vi "analyzepreLabel.vi"(0 "input_str_preLabel":string="L7KQF003-SD-R1510100004", 1 "input_int_SNNum":i32) -> (2 "show_bool_legal":bool, 3 "show_time_date":timestamp, 4 "show_str_message":string)   [LabVIEW 2011]
panel:
  out "midVar_str_yymmdd":string
  # "L7KQF003-SD-R1510100004\n    151010\nLR151010000001\n    101000\nLR15"
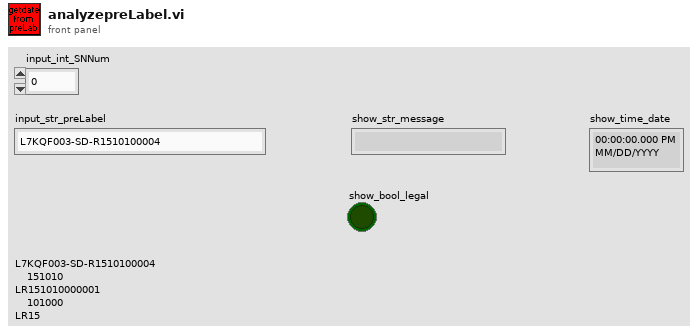
[diagram p1: front panel]
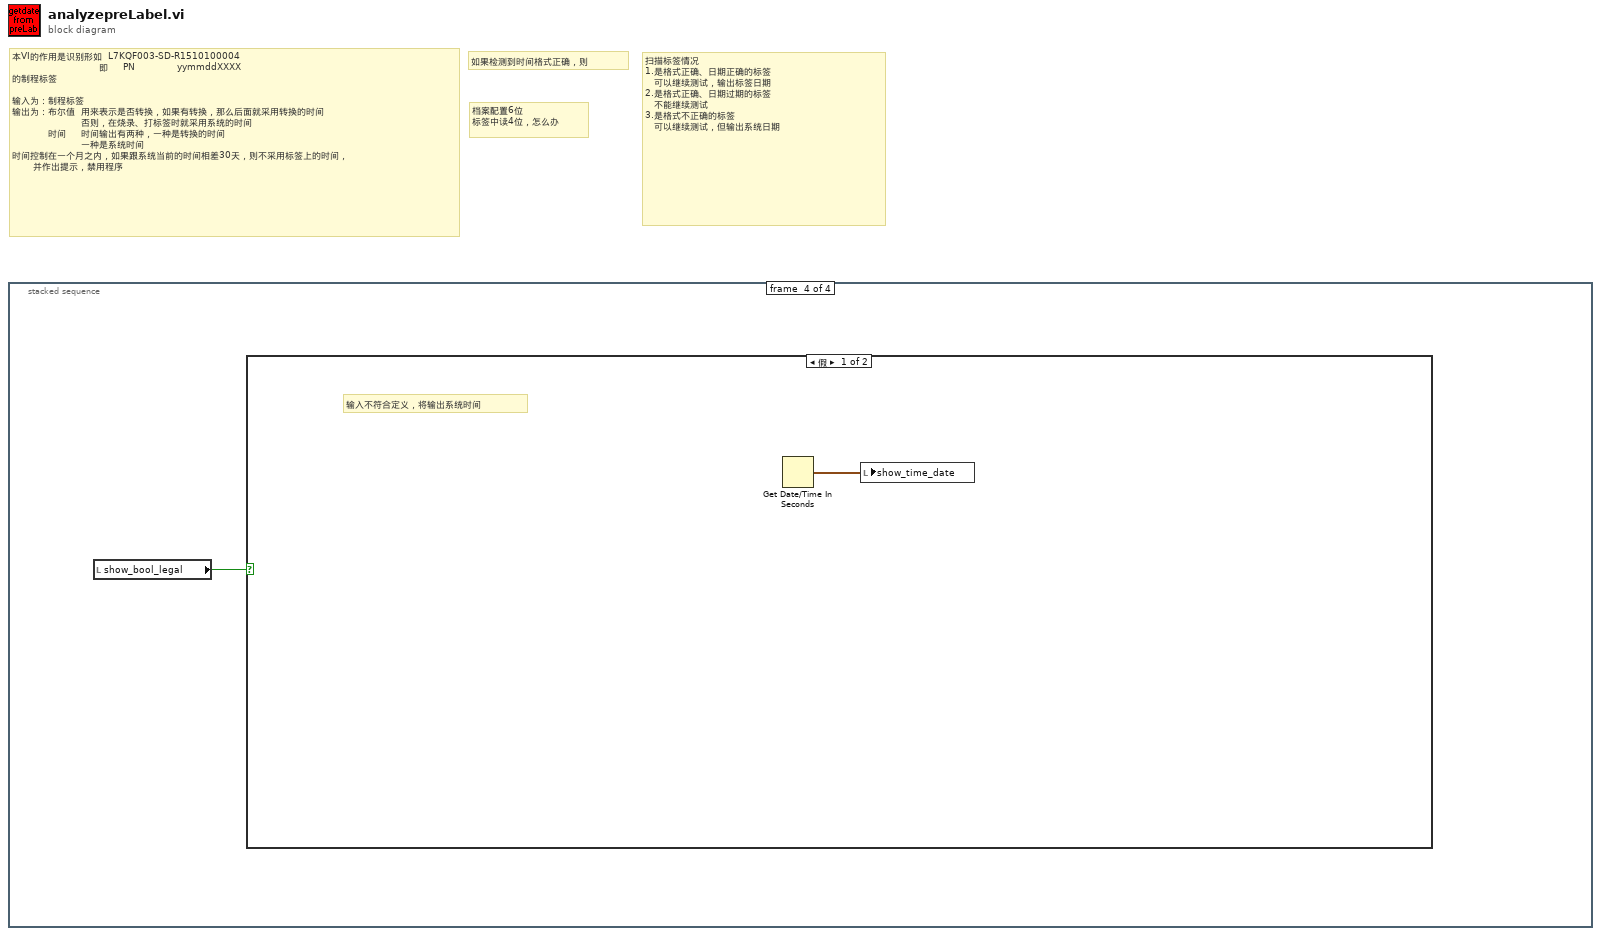
[diagram p0: block diagram]
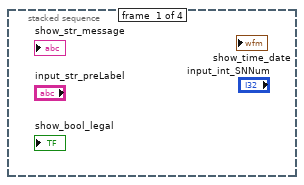
[diagram p2: hidden frame]
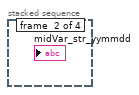
[diagram p3: hidden frame]
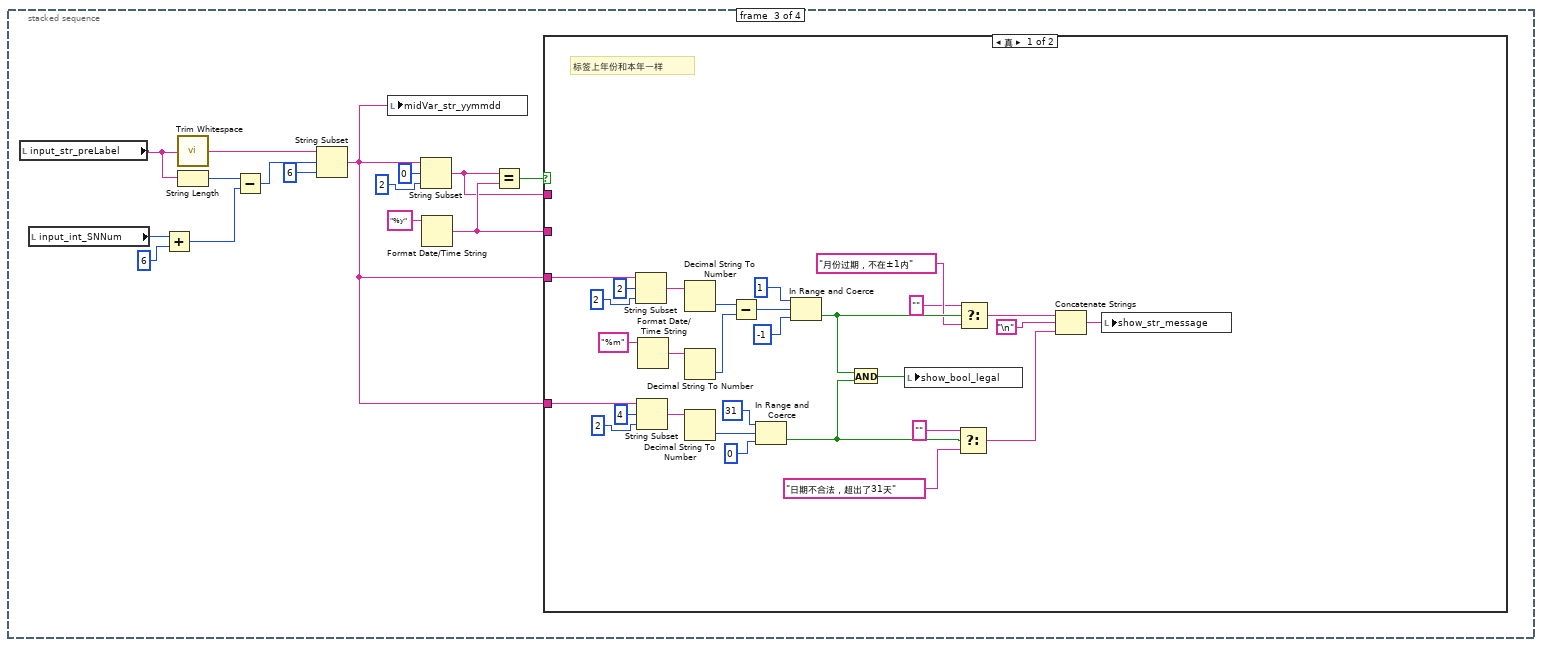
[diagram p4: hidden frame]
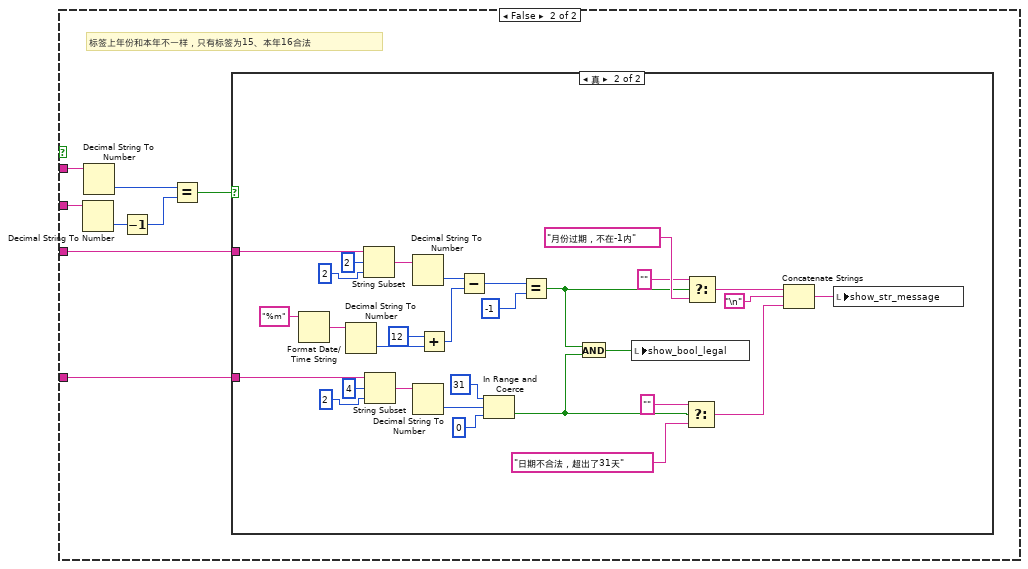
[diagram p5: hidden frame]
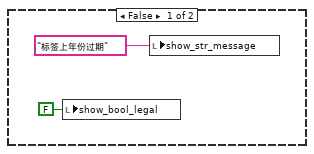
[diagram p6: hidden frame]
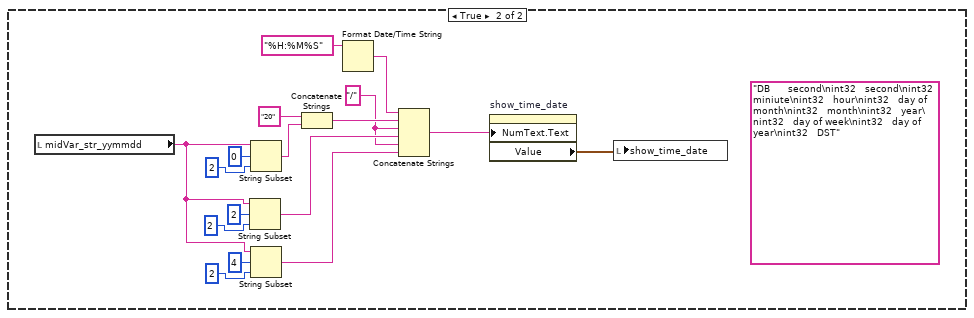
[diagram p7: hidden frame]
diagram:
  # "扫描标签情况\n1.是格式正确、日期正确的标签\n   可以继续测试，输出标签日期\n2.是格式正确、日期过期的标签\n   不能继续测试\n3.是格式不正确的标签\n   可以继续测试，但输出系统日期"
  # "档案配置6位\n标签中读4位，怎么办"
  # "如果检测到时间格式正确，则"
  # "本VI的作用是识别形如  L7KQF003-SD-R1510100004\n                             即     PN              yymmddXXXX\n的制程标签\n\n输入为：制程标签\n输出为：布尔值  用来表示是否转换，如果有转换，那么后面就采用转换的时间\n                       否则，在烧录、打标签时就采用系统的时间\n            时间     时间输出有两种，一种是转换的时间\n                       一种是系统时间\n时间控制在一个月之内，如果跟系统当前的时间相差30天，则不采用标签上的时间，\n       并作出提示，禁用程序"
  n1 = stacked-sequence {
    frame #0 {
    }
    frame #1 {
    }
    frame #2 {
      n2 = local read "input_str_preLabel"() -> (w5:string)
      n3 = local read "input_int_SNNum"() -> (w3:i32)
      n4 = Add(x=w3, y=6) -> (x+y=w1:i32)
      n5 = call <vilib>:"Trim Whitespace.vi"("string"=w5) -> ("trimmed string"=w15:string)  [unwired: 1 in]
      n6 = String Length(string=w5) -> (length=w14:i32)
      n7 = Subtract(x=w14, y=w1) -> (x-y=w13:i32)
      n8 = String Subset(string=w15, offset (0)=w13, length (rest)=6 ("长度（剩余）")) -> (substring=w4:string)
      n9 = local write "midVar_str_yymmdd"(w4) -> ()
      n10 = String Subset(string=w4, offset (0)=0 ("偏移量(0)"), length (rest)=2 ("长度（剩余）")) -> (substring=w6:string)
      n11 = Format Date/Time String(time format string (%c)="%y" ("时间格式字符串(%c)")) -> (date/time string=w7:string)  [unwired: 2 in]
      n12 = Equal?(x=w6, y=w7) -> (x = y?=w8:bool)
      n13 = case shown="真" w8 {
        tunnel: w4 -> [w41 w52]
        tunnel: w4 -> [w31 w51]
        tunnel: w7 -> [_ w50]
        tunnel: w6 -> [_ w48]
        frame True {
          # "标签上年份和本年一样"
          n14 = String Subset(string=w41, offset (0)=2 ("偏移量(0)"), length (rest)=2 ("长度（剩余）")) -> (substring=w40:string)
          n15 = String Subset(string=w31, offset (0)=4 ("偏移量(0)"), length (rest)=2 ("长度（剩余）")) -> (substring=w30:string)
          n16 = Format Date/Time String(time format string (%c)="%m" ("时间格式字符串(%c)")) -> (date/time string=w39:string)  [unwired: 2 in]
          n17 = Decimal String To Number(string=w40) -> (number=w38:i32)  [unwired: 2 in, 1 out]
          n18 = Decimal String To Number(string=w39) -> (number=w37:i32)  [unwired: 2 in, 1 out]
          n19 = Decimal String To Number(string=w30) -> (number=w29:i32)  [unwired: 2 in, 1 out]
          n20 = Subtract(x=w38, y=w37) -> (x-y=w36:i32)
          n21 = In Range and Coerce(upper limit=31 ("上限"), x=w29, lower limit=0 ("下限")) -> (In Range?=w25:bool)  [unwired: 1 out]
          n22 = In Range and Coerce(upper limit=1 ("上限"), x=w36, lower limit=-1 ("下限")) -> (In Range?=w26:bool)  [unwired: 1 out]
          n23 = And(x=w26, y=w25) -> (x .and. y?=w16:bool)
          n24 = local write "show_bool_legal"(w16) -> ()
          n25 = Select(t="", s=w25, f="日期不合法，超出了31天") -> (s? t:f=w18:string)
          n26 = Select(t="", s=w26, f="月份过期，不在±1内") -> (s? t:f=w20:string)
          n27 = Concatenate Strings(w20, "\n", w18) -> (w17:string)
          n28 = local write "show_str_message"(w17) -> ()
        }
        frame False {
          # "标签上年份和本年不一样，只有标签为15、本年16合法"
          n29 = Decimal String To Number(string=w50) -> (number=w49:i32)  [unwired: 2 in, 1 out]
          n30 = Decimal String To Number(string=w48) -> (number=w47:i32)  [unwired: 2 in, 1 out]
          n31 = Decrement(x=w49) -> (x-1=w46:i32)
          n32 = Equal?(x=w47, y=w46) -> (x = y?=w45:bool)
          n33 = case shown="真" w45 {
            tunnel: w52 -> [_ w81]
            tunnel: w51 -> [_ w75]
            frame False {
              n34 = local write "show_bool_legal"(FALSE ("show_bool_legal")) -> ()
              n35 = local write "show_str_message"("标签上年份过期" ("show_str_message")) -> ()
            }
            frame True {
              n36 = Format Date/Time String(time format string (%c)="%m" ("时间格式字符串(%c)")) -> (date/time string=w79:string)  [unwired: 2 in]
              n37 = Decimal String To Number(string=w79) -> (number=w60:i32)  [unwired: 2 in, 1 out]
              n38 = String Subset(string=w81, offset (0)=2 ("偏移量(0)"), length (rest)=2 ("长度（剩余）")) -> (substring=w80:string)
              n39 = String Subset(string=w75, offset (0)=4 ("偏移量(0)"), length (rest)=2 ("长度（剩余）")) -> (substring=w74:string)
              n40 = Decimal String To Number(string=w80) -> (number=w78:i32)  [unwired: 2 in, 1 out]
              n41 = Decimal String To Number(string=w74) -> (number=w73:i32)  [unwired: 2 in, 1 out]
              n42 = Add(x=12, y=w60) -> (x+y=w61:i32)
              n43 = Subtract(x=w78, y=w61) -> (x-y=w58:i32)
              n44 = In Range and Coerce(upper limit=31 ("上限"), x=w73, lower limit=0 ("下限")) -> (In Range?=w70:bool)  [unwired: 1 out]
              n45 = Equal?(x=w58, y=-1 ("下限")) -> (x = y?=w56:bool)
              n46 = And(x=w56, y=w70) -> (x .and. y?=w55:bool)
              n47 = local write "show_bool_legal"(w55) -> ()
              n48 = Select(t="", s=w70, f="日期不合法，超出了31天") -> (s? t:f=w63:string)
              n49 = Select(t="", s=w56, f="月份过期，不在-1内") -> (s? t:f=w65:string)
              n50 = Concatenate Strings(w65, "\n", w63) -> (w62:string)
              n51 = local write "show_str_message"(w62) -> ()
            }
          }
        }
      }
    }
    frame #3 {
      n52 = local read "show_bool_legal"() -> (w85:bool)
      n53 = case shown="假" w85 {
        frame False {
          # "输入不符合定义，将输出系统时间"
          n54 = Get Date/Time In Seconds() -> (seconds since 1Jan1904=w86:timestamp)
          n55 = local write "show_time_date"(w86) -> ()
        }
        frame True {
          w92 = "/"
          (unwired) "DB      second\nint32   second\nint32   miniute\nint32   hour\nint32   day of month\nint32   month\nint32   year\nint32   day of week\nint32   day of year\nint32   DST"
          n56 = local read "midVar_str_yymmdd"() -> (w95:string)
          n57 = String Subset(string=w95, offset (0)=2 ("偏移量(0)"), length (rest)=2 ("长度（剩余）")) -> (substring=w93:string)
          n58 = String Subset(string=w95, offset (0)=0 ("偏移量(0)"), length (rest)=2 ("长度（剩余）")) -> (substring=w100:string)
          n59 = String Subset(string=w95, offset (0)=4 ("偏移量(0)"), length (rest)=2 ("长度（剩余）")) -> (substring=w91:string)
          n60 = Concatenate Strings("20", w100) -> (w94:string)
          n61 = Format Date/Time String(time format string (%c)="%H:%M%S" ("时间格式字符串(%c)")) -> (date/time string=w89:string)  [unwired: 2 in]
          n62 = Concatenate Strings(w89, w94, w92, w93, w92, w91) -> (w88:string)
          n63 = property on="show_time_date" class="AbsTime (严格)"("NumText.Text"=w88) -> ("Value"=w87:timestamp)  [unwired: 2 in, 2 out]
          n64 = local write "show_time_date"(w87) -> ()
        }
      }
    }
  }
